vi "_Update TIC Property.vi"(10 "Current Data":T2={"Scan#"=0, "Run Time (mS)"=0, "TIC X"=[], "TIC Y"=[], "MassRange"=[], "Fixed Mass (amu)"=1.0, "Method"={"StartT(mS)"=0, "#Cycles"=0, "PauseT(uS)"=0, "ScanType"=0, "Polarity"=0, "FixedMass"=0.0, "DelayT(mS)"=0, "Active Ch"=[], "Mass Range"=[]}} {"Method"."Mass Range"."Res" items=["High/High", "Medium/Medium", "Low/Low", "High/Medium", "High/Low", "Medium/High", "Medium/Low", "Low/High", "Low/Medium"]}) -> (0 "Run Mode":T1, 1 "YMax":dbl, 2 "TIC Data":cluster{"TIC X":dbl[], "Data in cps":dbl[]}[](array[cluster]), 3 "YTitle":string, 4 "Q2DC Pol":bool, 5 "Q1DC Pol":bool, 6 "MCA":bool, 7 "XTitle":string)   [LabVIEW 2012]
uses:
  Type/_Current Data.ctl
  Type/_XML Expt.ctl
  Type/_XML Lens.ctl
  Type/_Mass Range Property.ctl
  Type/_Mass Range Parameters.ctl
  Type/_RT Res Type.ctl
  Type/_Run Mode.ctl
  Type/_Run Module.ctl
  Configuration/_Global Configuration.vi
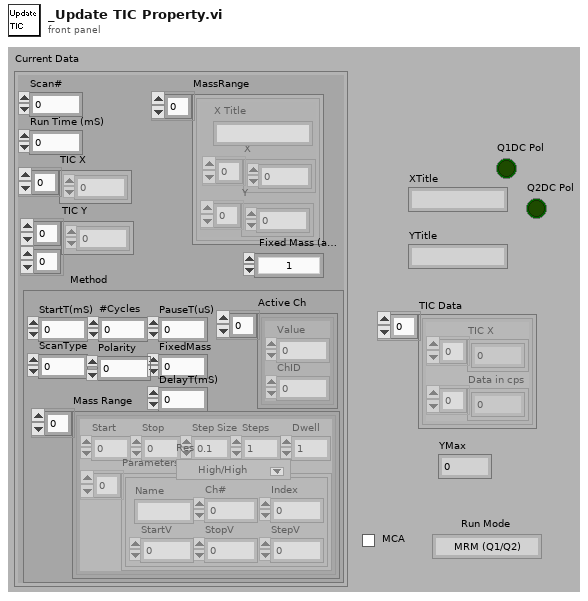
[diagram p1: front panel]
types:
  T1 = typedef "_Run Mode.ctl" = enum16{"MRM (Q1/Q2)", "Q1 Scan", "Q1 SRM", "Q2 Scan", "Q2 SRM", "Product Scan", "Precursor Scan", "Neutral Loss", "Neutral Gain"}
  T2 = typedef "_Current Data.ctl" = cluster{"Scan#":i32, "Run Time (mS)":i32, "TIC X":dbl[], "TIC Y":dbl[][], "MassRange":cluster{"X Title":string, "X":dbl[], "Y":i32[]}[], "Fixed Mass (amu)":dbl, "Method":T3}
  T3 = typedef "_XML Expt.ctl" = cluster{"StartT(mS)":i32, "#Cycles":i32, "PauseT(uS)":i32, "ScanType":i32, "Polarity":u8, "FixedMass":dbl, "DelayT(mS)":i32, "Active Ch":T4[], "Mass Range":T5[]}
  T4 = typedef "_XML Lens.ctl" = cluster{"Value":dbl, "ChID":u8}
  T5 = typedef "_Mass Range Property.ctl" = cluster{"Start":dbl, "Stop":dbl, "Step Size":dbl, "Steps":i32, "Dwell":dbl, "Parameters":T6[], "Res":T7}
  T6 = typedef "_Mass Range Parameters.ctl" = cluster{"Name":string, "Ch#":u8, "StartV":dbl, "StopV":dbl, "StepV":dbl, "Index":u8}
  T7 = typedef "_RT Res Type.ctl" = u16
  T8 = typedef "_Run Module.ctl" = u16
  T9 = typedef "_Lens Property.ctl" = cluster{"Scan Type":u8, "Scans":i32, "Time 1":dbl, "Time 2":dbl, "Value 1":dbl, "Value 2":dbl, "Step Size":dbl}
  T10 = cluster{"Lenses":T9[], "Mass Ranges":T5[], "Acquire":bool, "MCA":bool, "Q1DC EN":bool, "Q1 POL":bool, "Q3 POL":bool, "Q1 RF  EN":bool, "Averaging":bool, "Log Scale":bool, "CPS":bool, "Unit":bool, "Data Path":path, "Run Mode":T1, "Fixed Mass (amu)":dbl, "Q3DC EN":bool, "Q3 RF  EN":bool, "Negative":bool}
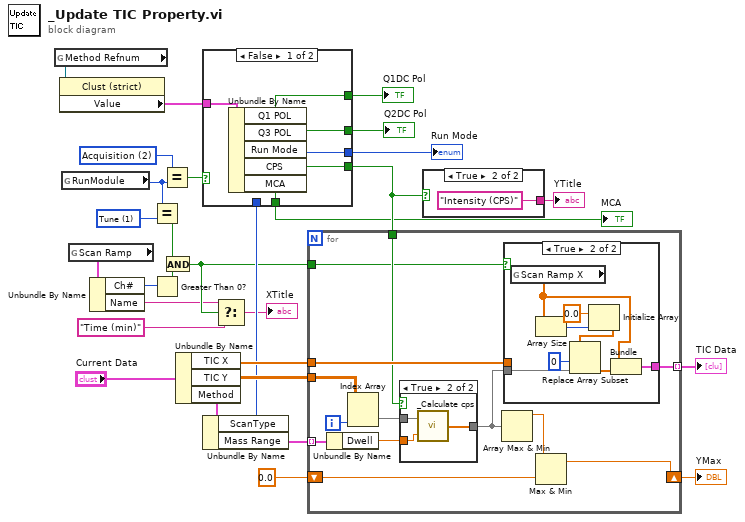
[diagram p0: block diagram]
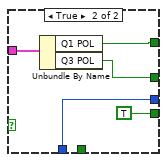
[diagram p2: hidden frame]
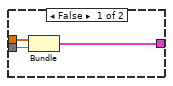
[diagram p3: hidden frame]
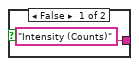
[diagram p5: hidden frame]
diagram:
  w13 = T8 1 items=["Diagnostics", "Tune", "Acquisition"] ("y")
  w15 = T8 2 items=["Diagnostics", "Tune", "Acquisition"] ("y")
  n1 = global read "_Global Configuration.vi" "Method Refnum"() -> (w4:refnum<vi>)
  n2 = property class="Clust (strict)"(reference=w4) -> ("Value"=w3:T10)  [unwired: 1 in, 2 out]
  n3 = global read "_Global Configuration.vi" "RunModule"() -> (w14:T8)
  n4 = global read "_Global Configuration.vi" "Scan Ramp"() -> (w12:T6)
  n5 = Unbundle By Name(w12) -> ("Ch#"=w11:u8, "Name"=w6:string)
  n6 = Equal?(x=w14, y=w13) -> (x = y?=w10:bool)
  n7 = Greater Than 0?(x=w11) -> (x > 0?=w9:bool)
  n8 = Equal?(x=w15, y=w14) -> (x = y?=w17:bool)
  n9 = And(x=w10, y=w9) -> (x .and. y?=w8:bool)
  n10 = Unbundle By Name("Current Data") -> ("TIC X"=w28:dbl[], "TIC Y"=w27:dbl[][], "Method"=w26:T3)
  n11 = Unbundle By Name(w26) -> ("ScanType"=w16:i32, "Mass Range"=w18:T5[])
  n12 = case shown="False" w17 {
    tunnel: [w35 TRUE ("CPS")] -> w25
    tunnel: [w34 w40] -> w20
    tunnel: [w33 _] -> w19
    tunnel: w16 -> [_ w40]
    tunnel: w3 -> [w32 w38]
    tunnel: [w31 w37] -> w2
    tunnel: [w30 w36] -> w1
    frame False {
      n13 = Unbundle By Name(w32) -> ("Q1 POL"=w31:bool, "Q3 POL"=w30:bool, "Run Mode"=w34:T1, "CPS"=w35:bool, "MCA"=w33:bool)
    }
    frame True {
      n14 = Unbundle By Name(w38) -> ("Q1 POL"=w37:bool, "Q3 POL"=w36:bool)
    }
  }
  "Run Mode" <- w20
  "MCA" <- w19
  "Q1DC Pol" <- w2
  "Q2DC Pol" <- w1
  n15 = Select(t=w6, s=w8, f="Time (min)") -> (s? t:f=→"XTitle":string)
  n16 = for {
    tunnel: w28 -> [w53]
    tunnel: w27 -> [w52]
    tunnel: [w50] -> w22 mode=indexing
    tunnel: w18 -> [w49] mode=indexing
    tunnel: w25 -> [w48]
    shift-right: [w43] -> w21
    shift-left: 0.0 -> [w45]
    tunnel: w8 -> [w41]
    i -> [w51]
    n17 = Unbundle By Name(w49) -> ("Dwell"=w47:dbl)
    n18 = Index Array(array=w52, index (col)=w51) -> (element=w42:dbl[])  [unwired: 1 in]
    n19 = case shown="True" w48 {
      tunnel: w42 -> [w65 w68]
      tunnel: w47 -> [_ w67]
      tunnel: [w65 w66] -> w46
      frame False {
      }
      frame True {
        n20 = call "_Calculate cps.vi"("Dwell (mS)"=w67, "Raw Counts"=w68) -> ("Data in cps"=w66:dbl[])
      }
    }
    n21 = Array Max & Min(array=w46) -> (max value=w44:dbl)  [unwired: 3 out]
    n22 = case shown="True" w41 {
      tunnel: w53 -> [w56 _]
      tunnel: [w55 w57] -> w50
      tunnel: w46 -> [w54 w60]
      frame False {
        n23 = Bundle("TIC X"=w56, "Data in cps"=w54) -> (w55:cluster{"TIC X":dbl[], "Data in cps":dbl[]})  [unwired: 1 out]
      }
      frame True {
        n24 = global read "_Global Configuration.vi" "Scan Ramp X"() -> (w58:dbl[])
        n25 = Array Size(array=w58) -> (size(s)=w63:i32)
        n26 = Initialize Array(0.0 ("element"), w63) -> (w62:dbl[])
        n27 = Replace Array Subset(array=w62, new element=w60, index=0) -> (w59:dbl[])
        n28 = Bundle("Scan Ramp X"=w58, w59) -> (w57:cluster{"Scan Ramp X":dbl[], dbl[]})  [unwired: 1 out]
      }
    }
    n29 = Max & Min(x=w44, y=w45) -> (max(x,y)=w43:dbl)  [unwired: 1 out]
  }
  "TIC Data" <- w22
  "YMax" <- w21
  n30 = case shown="True" w25 {
    tunnel: ["Intensity (Counts)" "Intensity (CPS)"] -> w23
    frame False {
    }
    frame True {
    }
  }
  "YTitle" <- w23
